vi "SutterController2.vi"() -> ()   [LabVIEW 2012]
panel:
  out "Numeric":i32
  in  "go":bool
  in  "position":dbl[](array[numeric])
  out "Array":dbl[](array[numeric])
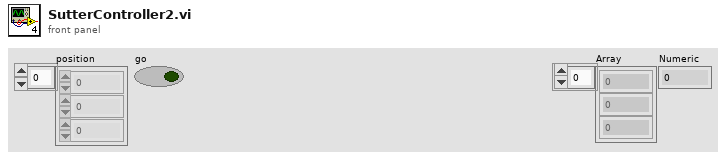
[diagram p1: front panel]
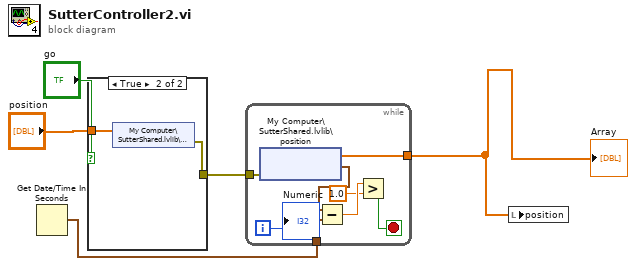
[diagram p0: block diagram]
diagram:
  n1 = Get Date/Time In Seconds() -> (seconds since 1Jan1904=w1:timestamp)
  n2 = case shown="True" "go" {
    tunnel: "position" -> [_ w7]
    tunnel: [_ w6] -> w3
    frame False {
    }
    frame True {
      n3 = shared-variable "My Computer\\SutterShared.lvlib\\position"(w7) -> (error out=w6:errorcluster)  [unwired: 1 in]
    }
  }
  n4 = while {
    tunnel: [w15] -> w4
    tunnel: w3 -> [w14]
    tunnel: w1 -> [w12]
    i -> [w8]
    stop <- w9 stop-if-true
    n5 = shared-variable "My Computer\\SutterShared.lvlib\\position"(error in=w14) -> (w15:dbl[], w13:timestamp)  [unwired: 1 out]
    n6 = Subtract(x=w13, y=w12) -> (x-y=w11:dbl)
    n7 = Greater?(x=w11, y=1.0) -> (0:w9:bool)
    "Numeric" <- w8
  }
  "Array" <- w4
  n8 = local write "position"(w4) -> ()
